vi "_Test Dashed Test Method.vi"(8 "error in (no error)":errorcluster, 11 "Dummy Test Case in":refnum<class "_Dashed Dummy.lvclass">) -> (0 "error out":errorcluster, 3 "Dummy Test Case out":refnum<class "_Dashed Dummy.lvclass">)   [LabVIEW 2020, in "_Dashed Dummy.lvclass"]
uses:
  _Dashed Dummy.lvclass
  C:/git/astemes-lunit/source/API/LUnit Test Case/LUnit Test Case.lvclass
  source/API/LUnit Test Case/LUnit Test Case.lvclass/LUnit Test Case.ctl
  source/API/LUnit Test Case/Private/Append Fail Result.vi
  _Dashed Dummy.lvclass/_Dashed Dummy.ctl
  source/API/LUnit Test Case/LUnit Test Case.lvclass
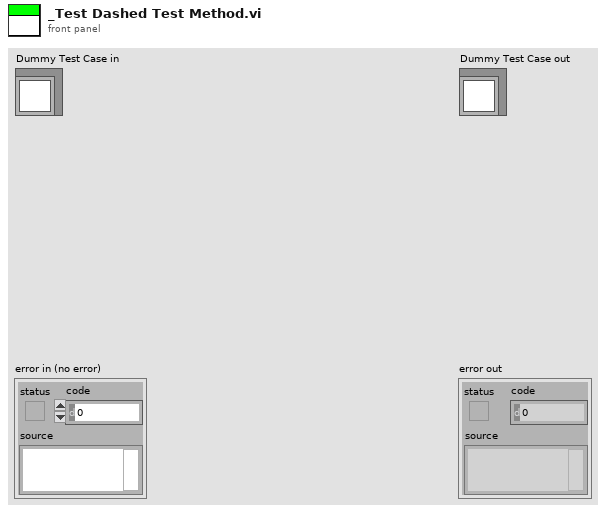
[diagram p1: front panel]
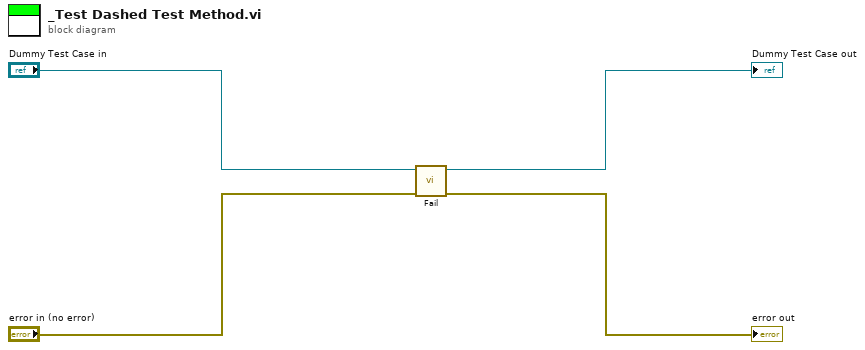
[diagram p0: block diagram]
diagram:
  n1 = call "Fail.vi"("error in (no error)"="error in (no error)", "LUnit Test Case In"="Dummy Test Case in") -> ("error out"=→"error out":errorcluster, "LUnit Test Case Out"=→"Dummy Test Case out":refnum<class "_Dashed Dummy.lvclass">)  [unwired: 8 in]
